vi "Demo.vi"() -> ()   [LabVIEW 2020]
uses:
  GPIO Channel.ctl
panel:
  out "Read State":bool
  out "error out":errorcluster
  in  "Write State":bool
  in  "Channel Write":T1
  in  "Write":bool
  in  "Channel to Read":T1
  in  "Read":bool
  # "Read"
  # "Write"
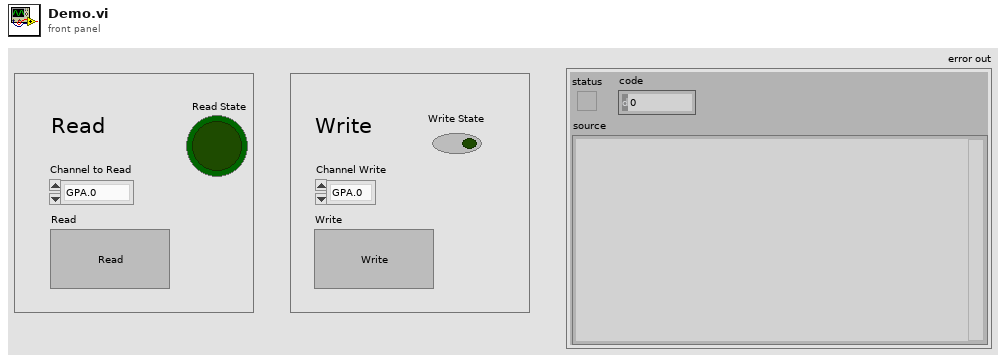
[diagram p1: front panel]
types:
  T1 = typedef "GPIO Channel.ctl" = enum16{"GPA.0", "GPA.1", "GPA.2", "GPA.3", "GPA.4", "GPA.5", "GPA.6", "GPA.7", "GPB.0", "GPB.1", "GPB.2", "GPB.3", "GPB.4", "GPB.5", "GPB.6", "GPB.7"}
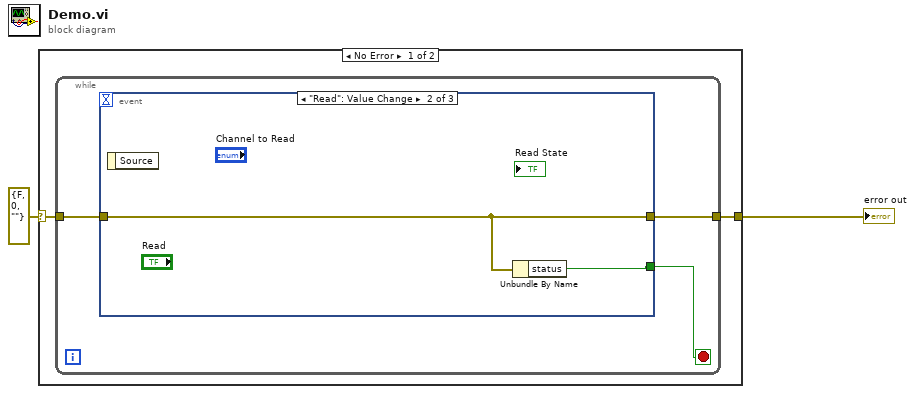
[diagram p0: block diagram]
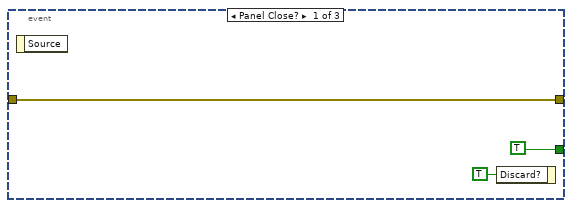
[diagram p2: hidden frame]
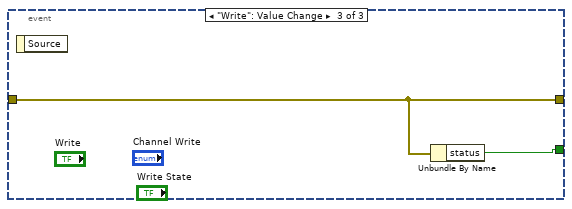
[diagram p3: hidden frame]
diagram:
  n1 = case shown="No Error" errorcluster {"status"=FALSE, "code"=0, "source"=""} ("error IO") {
    selector: errorcluster {"status"=FALSE, "code"=0, "source"=""} ("error IO") -> [w4 w15]
    tunnel: [w3 w15] -> w2
    frame No Error {
      n2 = while {
        tunnel: w4 -> [w7]
        tunnel: [w5] -> w3
        stop <- w6 stop-if-true
        n3 = event shown="[1] \"Read\": Value Change" {
          selector: _ -> [_ _ _]
          dyn-events: _ -> [_ _ _]
          timeout: _ -> [_ _ _]
          tunnel: w7 -> [w8 w12 w14]
          tunnel: [TRUE w11 w13] -> w6
          tunnel: [w8 w12 w14] -> w5
          event Panel Close? {
            n4 = event-data() -> ()  [unwired: 1 in, 1 out]
            n5 = event-data("Discard?"=TRUE) -> ()  [unwired: 1 in, 1 out]
          }
          event "Read": Value Change {
            n6 = event-data() -> ()  [unwired: 1 in, 1 out]
            n7 = Unbundle By Name(w12) -> ("status"=w11:bool)
          }
          event "Write": Value Change {
            n8 = event-data() -> ()  [unwired: 1 in, 1 out]
            n9 = Unbundle By Name(w14) -> ("status"=w13:bool)
          }
        }
      }
    }
    frame Error {
    }
  }
  "error out" <- w2
